vi "Set BrowerComponentIndex.vi"(8 "error in (no error)":errorcluster, 10 "SymbolIndex":i32, 11 "BrowerComponent in":refnum<class "BrowerComponent.lvclass">) -> (0 "error out":errorcluster, 3 "BrowerComponent out":refnum<class "BrowerComponent.lvclass">)   [LabVIEW 2015, in "BrowerComponent.lvclass"]
uses:
  BrowerComponent.lvclass
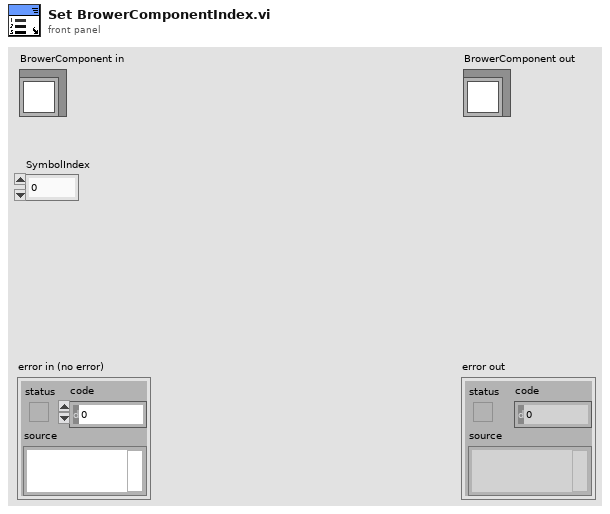
[diagram p1: front panel]
types:
  T1 = typedef "BrowerComponent.lvclass/ObjectAttributes.ctl" = cluster{"ComponentID":string, "SymbolIndex":i32, "ComponentName":string, "PartsOfComponent_dict":variant}
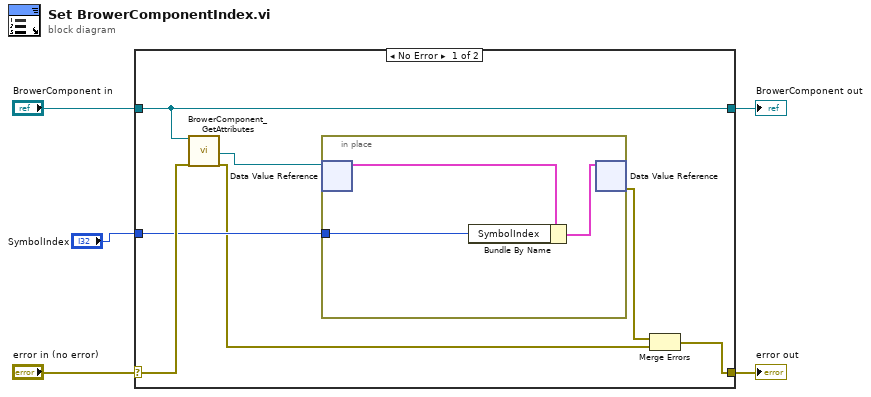
[diagram p0: block diagram]
diagram:
  n1 = case shown="No Error" "error in (no error)" {
    selector: "error in (no error)" -> [w11 w17]
    tunnel: [w8 w17] -> w4
    tunnel: [w12 w16] -> w2
    tunnel: "BrowerComponent in" -> [w12 w16]
    tunnel: "SymbolIndex" -> [w7 _]
    frame No Error {
      n2 = call "BrowerComponent_GetAttributes.vi"("reference in"=w12, "error in (no error)"=w11) -> ("DataRef"=w10:refnum<data-value>, "error out"=w6:errorcluster)  [unwired: 14 in, 2 out]
      n3 = in-place {
        in-place-border: w7 -> [w13]
        n4 = in-place-dvr #1(w10) -> (w15:T1)  [unwired: 1 out]
        n5 = Bundle By Name(cluster=w15, "SymbolIndex"=w13) -> (w14:T1)
        n6 = in-place-dvr #1(w14) -> (w9:errorcluster)  [unwired: 1 out]
      }
      n7 = Merge Errors(w9, w6) -> (w8:errorcluster)
    }
    frame Error {
    }
  }
  "error out" <- w4
  "BrowerComponent out" <- w2
